vi "Call DQMH Get Event Info VI.vi"(8 "error in (no error)":errorcluster, 11 "ProjectItem in":refnum<vi>) -> (0 "error out":errorcluster, 2 "Event Name":string, 4 "VI Ref":refnum<vi>)   [LabVIEW 2017, in "Open DQMH Request Message Diagram.lvlib"]
uses:
  <vilib>/Utility/traverseref.llb/TRef TravTarget.ctl
  Open DQMH Request Message Diagram.lvlib
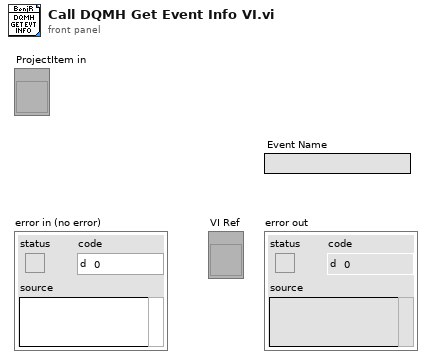
[diagram p1: front panel]
types:
  T1 = typedef "TRef TravTarget.ctl" = enum16{"FP", "BD", "Other"}
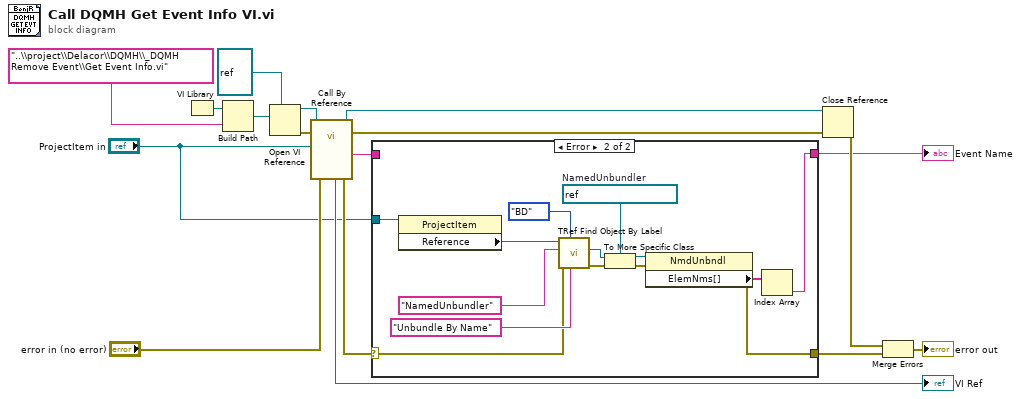
[diagram p0: block diagram]
diagram:
  n1 = VI Library() -> (path=w14:path)
  n2 = Build Path(base path=w14, name or relative path="..\\project\\Delacor\\DQMH\\_DQMH Remove Event\\Get Event Info.vi") -> (appended path=w13:path)
  n3 = Open VI Reference(type specifier VI Refnum (for type only)=refnum<vi> refnum, vi path=w13) -> (vi reference=w17:refnum<vi>, error out=w10:errorcluster)  [unwired: 4 in]
  n4 = call-by-ref "?"(reference=w17, error in=w10, 8:"error in (no error)"="error in (no error)", "ProjectItem in"="ProjectItem in") -> (reference out=w15:refnum<vi>, error out=w16:errorcluster, 0:"error out"=w5:errorcluster, "Event Name"=w4:string, "VI Ref"=→"VI Ref":refnum<vi>)  [unwired: 5 in, 2 out]
  n5 = case shown="Error" w5 {
    selector: w5 -> [w18 w21]
    tunnel: w4 -> [w19 _]
    tunnel: [w19 w23] -> w3
    tunnel: [w18 w22] -> w2
    tunnel: "ProjectItem in" -> [_ w20]
    frame No Error {
    }
    frame Error {
      w31 = refnum<vi> refnum  # NamedUnbundler
      n6 = property class="ProjectItem"(reference=w20) -> ("Reference"=w25:refnum<vi>)  [unwired: 1 in, 2 out]
      n7 = call <vilib>:"TRef Find Object By Label.vi"("Label"="Unbundle By Name" ("Class Name"), "Traverse Target"=TRef_TravTarget."BD", "error in (no error)"=w21, "Class Name"="NamedUnbundler", "VI Ref"=w25) -> ("error out"=w29:errorcluster, "Found Obj Ref"=w30:refnum<vi>)  [unwired: 3 in, 2 out]
      n8 = To More Specific Class(target class=w31, reference=w30, error in=w29) -> (specific class reference=w32:refnum<vi>, error out=w33:errorcluster)
      n9 = property class="NmdUnbndl"(reference=w32, error in=w33) -> (error out=w22:errorcluster, "ElemNms[]"=w26:string[])  [unwired: 1 out]
      n10 = Index Array(array=w26) -> (element=w23:string)  [unwired: 1 in]
    }
  }
  "Event Name" <- w3
  n11 = Close Reference(reference=w15, error in (no error)=w16) -> (error out=w12:errorcluster)
  n12 = Merge Errors(w12, w2) -> (→"error out":errorcluster)
